vi "dacTest.vi"() -> ()   [LabVIEW 2021]
panel:
  out "Y":dbl[](array[numeric])
  out "dt":dbl
  out "t0":timestamp
  out "Array 2":dbl[](array[numeric])
  in  "Array":dbl[](array[numeric])
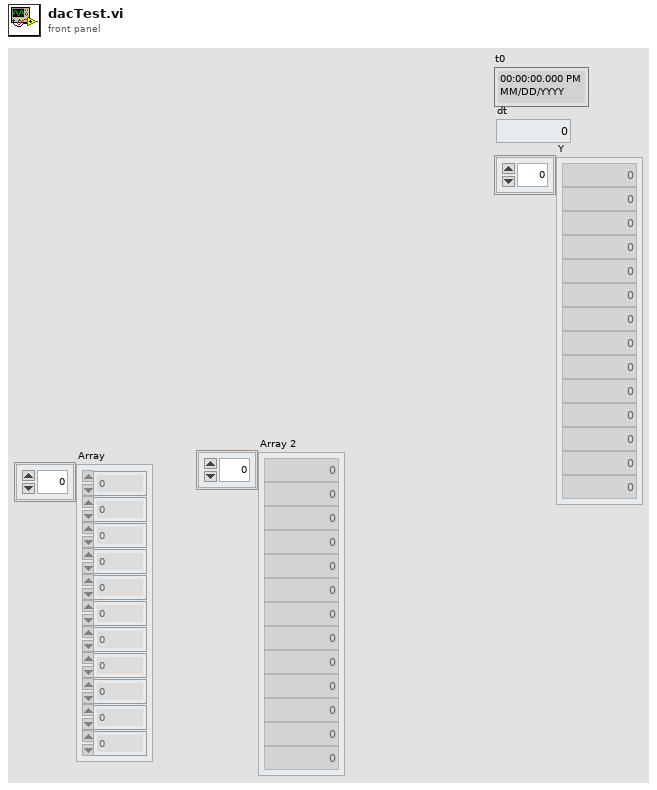
[diagram p1: front panel]
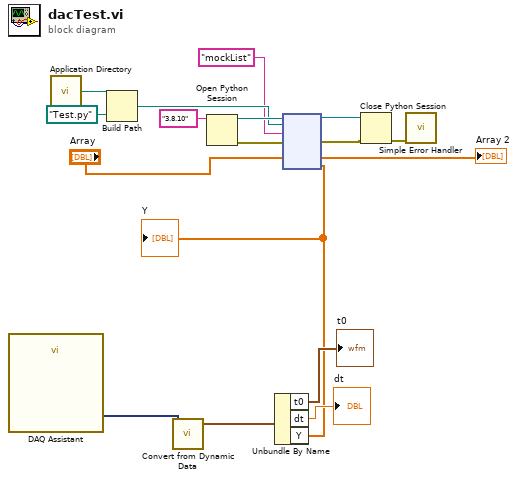
[diagram p0: block diagram]
diagram:
  n1 = call "DAQ Assistant"() -> ("data"=w5:dynamicdata)  [unwired: 17 in, 2 out]
  n2 = call <vilib>:"Application Directory.vi"() -> ("Application Directory"=w12:path)
  n3 = Build Path(base path=w12, name or relative path=path "Test.py") -> (appended path=w10:path)
  n4 = call "Convert from Dynamic Data"("Dynamic Data Type"=w5) -> ("Waveform"=w2:waveform(dbl))  [unwired: 3 in]
  n5 = Open Python Session(python version="3.8.10" ("Python version")) -> (session out=w17:refnum<k35>, error out=w16:errorcluster)  [unwired: 2 in]
  n6 = Unbundle By Name(w2) -> ("t0"=→"t0":timestamp, "dt"=→"dt":dbl, "Y"=w1:dbl[])
  "Y" <- w1
  n7 = node(w17, w10, "mockList" ("function name"), w16, "Array", w1) -> (w14:refnum<k35>, w15:errorcluster, →"Array 2":dbl[])  [unwired: 3 in, 2 out]
  n8 = Close Python Session(session in=w14, error in=w15) -> (11:w8:errorcluster)
  n9 = call <vilib>:"Simple Error Handler.vi"("error in (no error)"=w8) -> ()  [unwired: 4 in, 5 out]
